vi "writeDefectiveParts.vi"(0 "reference in":refnum<class "excelFile.lvclass">, 2 "data":string[][](array[string]), 5 "error in (no error)":errorcluster) -> (14 "reference out":refnum<class "excelFile.lvclass">, 19 "error out":errorcluster)   [LabVIEW 2016, in "excelFile.lvclass"]
uses:
  excelFile.lvclass
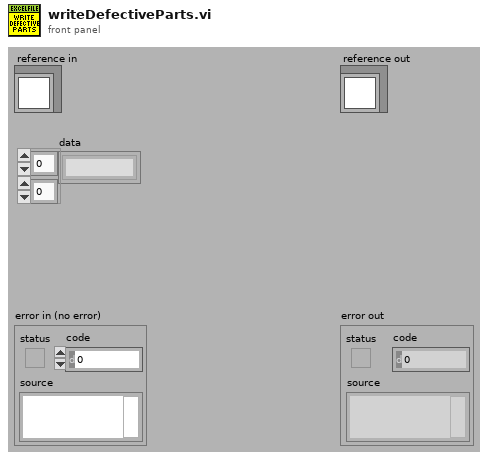
[diagram p1: front panel]
types:
  T1 = typedef "excelFile.lvclass/ObjectAttributesRef.ctl" = refnum<data-value>
  T2 = typedef "excelFile.lvclass/ObjectAttributes.ctl" = cluster{"MyAttribute":dbl, "path":string, "Refnum Excel":cluster{"Excel._Application":refnum<k7>, "Workbooks":refnum<k7>, "Open":refnum<k7>}, "data":string[][][], "save":bool, "fileType":T3, "rowsColor":u32[], "python_ref":refnum<class "python.lvclass">, "items_rows":i32[], "excel_range":i32[][], "TSR":cluster{"number":string, "TSR_path":path, "service_path":path, "email_to":string}, "excel_already_opened?":bool, "file_already_opened?":bool, "excel_protected_opened?":bool, "Refnum Cluster Worksheets":cluster{"Excel._Application":refnum<k7>, "Workbooks":refnum<k7>, "Open":refnum<k7>, "Worksheets":refnum<k7>, "Excel._Worksheet":refnum<k7>}, "#_rows_defective":i32, "#_rows_spare":i32}
  T3 = typedef "excelFile.lvclass/fileType.ctl" = enum16{"devices", "items", "partsTracking", "TSR"}
  T4 = cluster{"Excel._Application":refnum<k7>, "Workbooks":refnum<k7>, "Open":refnum<k7>, "Worksheets":refnum<k7>, "Excel._Worksheet":refnum<k7>}
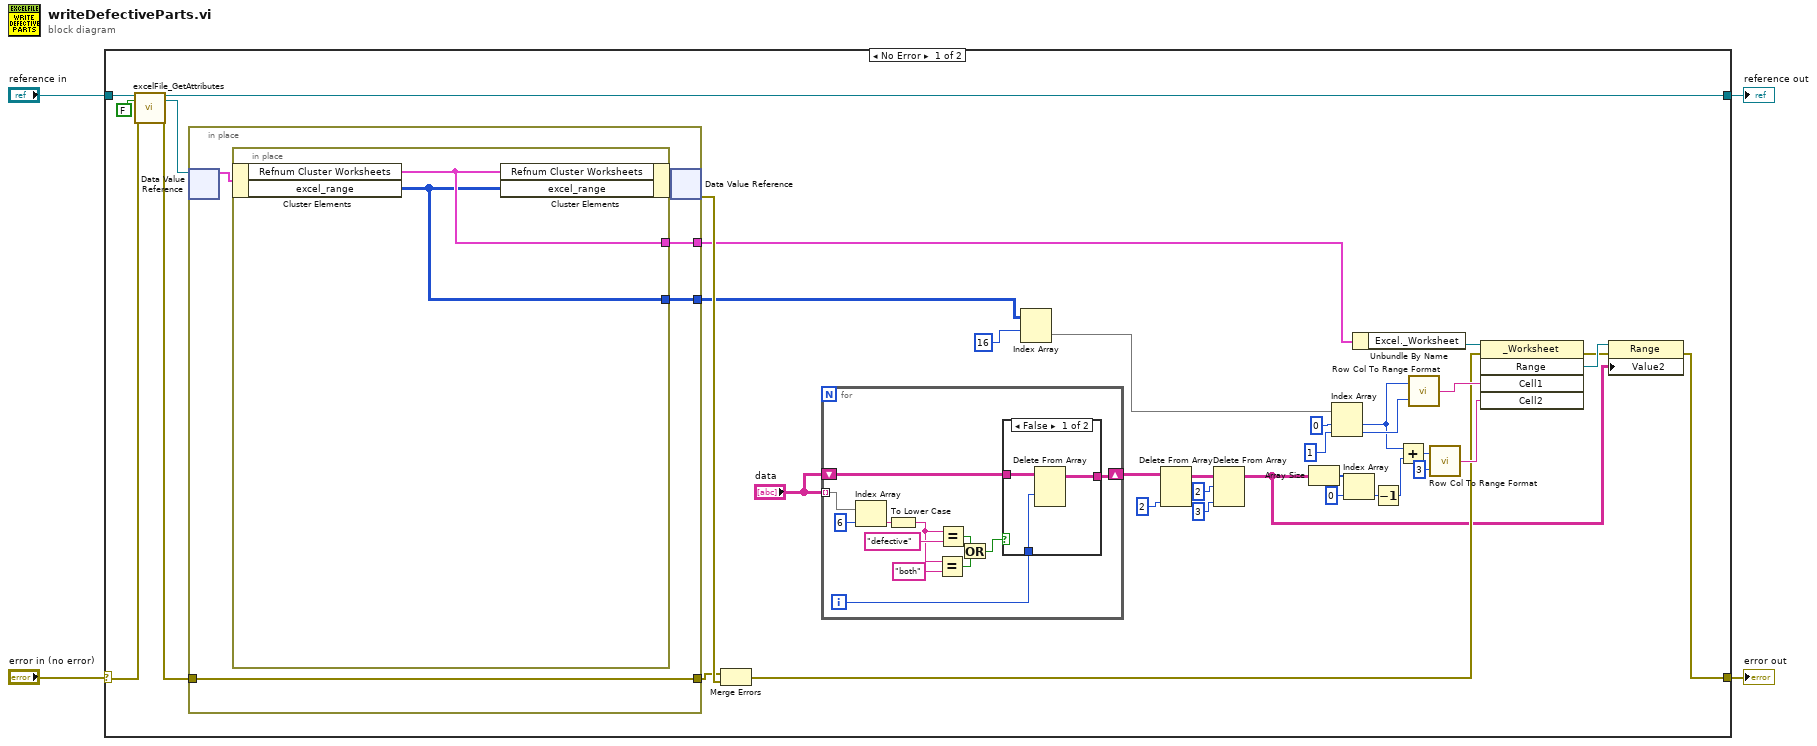
[diagram p0: block diagram]
diagram:
  n1 = case shown="No Error" "error in (no error)" {
    selector: "error in (no error)" -> [w36 w65]
    tunnel: [w8 w65] -> w3
    tunnel: [w34 w64] -> w1
    tunnel: "reference in" -> [w38 w64]
    frame No Error {
      n2 = call "excelFile_GetAttributes.vi"("reference in"=w38, "return data? (T)"=FALSE, "error in (no error)"=w36) -> ("reference out"=w34:refnum<class "excelFile.lvclass">, "attributes ref"=w33:T1, "error out"=w35:errorcluster)  [unwired: 13 in, 1 out]
      n3 = in-place {
        in-place-border: w35 -> [w59]
        in-place-border: [w59] -> w39
        in-place-border: [w58] -> w11
        in-place-border: [w57] -> w10
        n4 = in-place-dvr #1(w33) -> (w60:T2)  [unwired: 1 out]
        n5 = in-place {
          in-place-border: [w63] -> w58
          in-place-border: [w62] -> w57
          n6 = in-place-cluster #2(w60) -> ("Refnum Cluster Worksheets"=w63:T4, "excel_range"=w62:i32[][])
          n7 = in-place-cluster #2("Refnum Cluster Worksheets"=w63, "excel_range"=w62) -> (w61:T2)
        }
        n8 = in-place-dvr #1(w61) -> (w40:errorcluster)  [unwired: 1 out]
      }
      n9 = Merge Errors(w39, w40) -> (w9:errorcluster)
      n10 = for {
        tunnel: "data" -> [w52] mode=indexing
        shift-right: [w48] -> w28
        shift-left: "data" -> [w50]
        i -> [w49]
        n11 = Index Array(array=w52, index=6) -> (element=w47:string)
        n12 = To Lower Case(string=w47) -> (all lower case string=w44:string)
        n13 = Equal?(x=w44, y="both") -> (x = y?=w42:bool)
        n14 = Equal?(x=w44, y="defective") -> (x = y?=w43:bool)
        n15 = Or(x=w43, y=w42) -> (x .or. y?=w41:bool)
        n16 = case shown="False" w41 {
          tunnel: w50 -> [w55 w56]
          tunnel: w49 -> [w54 _]
          tunnel: [w53 w56] -> w48
          frame False {
            n17 = Delete From Array(array=w55, index (row)=w54) -> (array with subset deleted=w53:string[][])  [unwired: 2 in, 1 out]
          }
          frame True {
          }
        }
      }
      n18 = Index Array(array=w10, index (row)=16) -> (element=w7:i32[])  [unwired: 1 in]
      n19 = Delete From Array(array=w28, index (col)=2 ("disabled index (col)")) -> (array with subset deleted=w27:string[][])  [unwired: 2 in, 1 out]
      n20 = Delete From Array(array=w27, length=2 ("disabled index (col)"), index (col)=3 ("disabled index (col)")) -> (array with subset deleted=w5:string[][])  [unwired: 1 in, 1 out]
      n21 = Array Size(array=w5) -> (size(s)=w19:i32[])
      n22 = Index Array(array=w7, index #1=0 ("index"), index #2=1 ("index")) -> (element #1=w13:i32, element #2=w26:i32)
      n23 = Index Array(array=w19, index=0) -> (element=w15:i32)
      n24 = Unbundle By Name(w11) -> ("Excel._Worksheet"=w23:refnum<k7>)
      n25 = Decrement(x=w15) -> (x-1=w12:i32)
      n26 = Add(x=w13, y=w12) -> (x+y=w14:i32)
      n27 = call <userlib>:"Row Col To Range Format.vi"("Column"=w26, "Row"=w13) -> ("Output String"=w20:string)
      n28 = call <userlib>:"Row Col To Range Format.vi"("Column"=3, "Row"=w14) -> ("Output String"=w17:string)
      n29 = invoke class="_Worksheet" method="Range"(reference=w23, error in=w9, "Cell1"=w20, "Cell2"=w17) -> (error out=w21:errorcluster, "Range"=w22:refnum<k7>)  [unwired: 1 in, 3 out]
      n30 = property class="Range"(reference=w22, error in=w21, "Value2"=w5) -> (error out=w8:errorcluster)  [unwired: 1 out]
    }
    frame Error {
    }
  }
  "error out" <- w3
  "reference out" <- w1
